vi "ReadTDMS.vi"() -> ()   [LabVIEW 2016, in "VCL_2_DSC.lvclass"]
uses:
  lvsrc/VCL_2_DSC.lvclass
panel:
  out "Waveform Graph":waveform(dbl)(graph)
  out "element":string
  in  "disabled index (col)":i32
  in  "file path":path
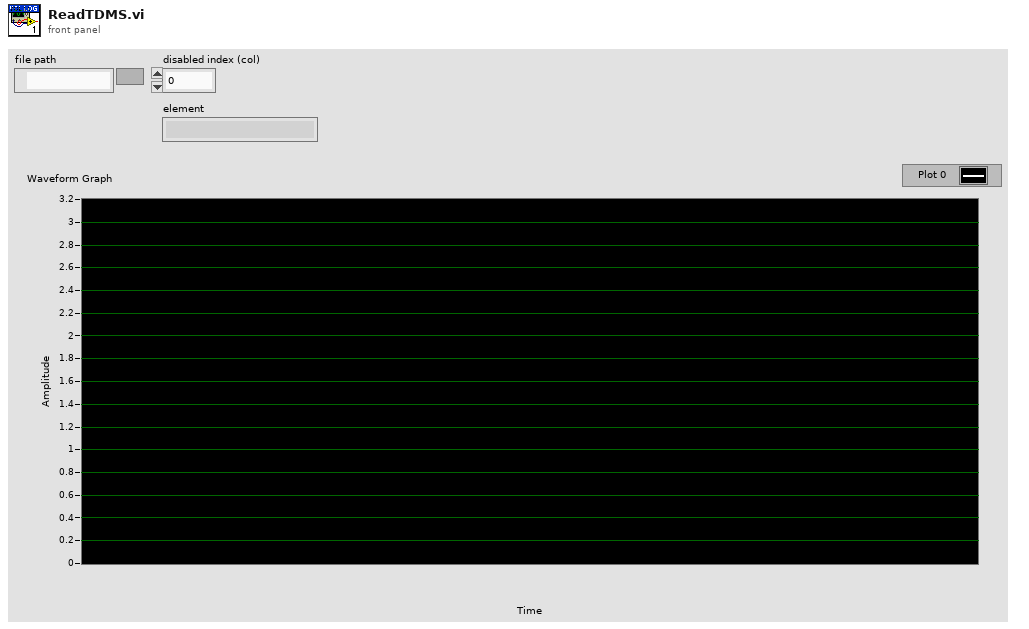
[diagram p1: front panel]
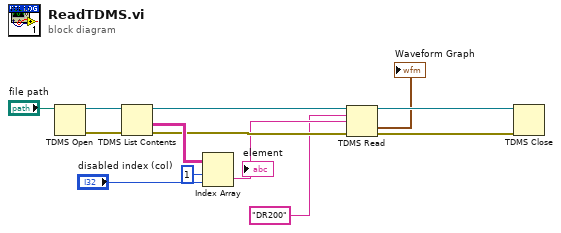
[diagram p0: block diagram]
diagram:
  n1 = TDMS Open(11:"file path") -> (0:w13:errorcluster, 3:w12:refnum<k34>)  [unwired: 6 in]
  n2 = TDMS List Contents(4:w13, 7:w12) -> (0:w7:errorcluster, 1:w10:string[][], 3:w6:refnum<k34>)  [unwired: 1 in, 1 out]
  n3 = Index Array(array=w10, index (row)=1, index (col)="disabled index (col)") -> (element=w5:string)
  "element" <- w5
  n4 = TDMS Read(0:w6, 5:"DR200" ("group name in"), 7:w5, 11:w7) -> (4:w2:refnum<k34>, 10:→"Waveform Graph":waveform(dbl), 15:w3:errorcluster)  [unwired: 4 in, 3 out]
  n5 = TDMS Close(8:w3, 11:w2) -> ()  [unwired: 2 out]
